vi "asyncAcq_occurenceRef_timeStamp.vi"(0 "reference":refnum<class "OSA.lvclass">, 5 "error in (no error)":errorcluster) -> (14 "duplicate reference":refnum<class "OSA.lvclass">, 15 "new spectrum":bool, 16 "new interferogram":bool, 18 "error":u32, 19 "error out":errorcluster)   [LabVIEW 2010, in "OSA.lvclass"]
doc: "Reads the contents of a <B>Thorlabs_OSA_64</B> object.\n\n[GOOP 1.0]"
uses:
  OSA.lvclass
panel:
  out "timeStamp interferogram":u32
  out "timeStamp spectrum":u32
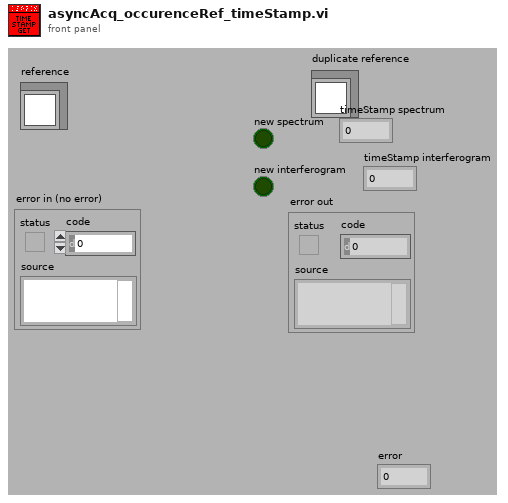
[diagram p1: front panel]
types:
  T1 = typedef "OSA.lvclass/ObjectAttributes.ctl" = cluster{"Stop":bool, "dataType":T2, "spectrometerIdx":u16, "buffer size interferogram":i32, "interferogram":cluster{"new":bool, "plot_x_ min":sgl, "plot_x_max":sgl, "plot_y_min":sgl, "plot_y_max":sgl, "Graph Intrfrgrm":T3, "timeStamp":u32, "signal (%)":dbl, "traces":cluster{"idx":u32, "broadBand":bool, "monoChromatic":bool, "peakToPeakSignal":dbl, "peakToPeakPos":dbl}[], "traces idx last":i32}, "spectrum":cluster{"new":bool, "plot_x_min":sgl, "plot_x_max":sgl, "plot_unit_x":T4, "plot_unit_y":T5, "plot_y_min":sgl, "plot_y_max":sgl, "Graph Spectrum":T3, "timeStamp":u32, "X_VAL_OPTIONS":enum16{"MIN_MAX", "ARRAY"}, "traces":cluster{"idx":u32}[], "traces idx last":i32}, "Thorlabs_OSA_64.lvclass:queue_action.ctlqueue ref":refnum<queue>, "action":T6, "plot zoom step":dbl, "buffer semaphore":T7, "acq stopped":bool, "dataType active":T2, "temperature (degr C)":sgl, "pressure (hPa)":sgl, "rel humidity (%)":sgl, "settings":cluster{"resolution":T8, "sensitivity":T9, "Average":bool, "average nr":u32, "apodisation":T10, "acq delay (ms)":u32, "airMesure":T11, "wmtr on":bool, "intfgrm_smooth_width":u16, "intfgrm_smooth_nrOfPasses":u16, "intfgrm_smooth":T12, "phaseCorrection":T13, "zeroFill":u8, "spectr_smooth":T12, "spectr_smooth_width":u16, "spectr_smooth_nrOfPasses":u16, "resolution (/cm)":sgl, "REF wavelength, (nm)":dbl, "gain_idx":u16, "gainAuto":bool, "gain_relative":dbl, "PD sensitivity mode":T14, "PD senseMode implemented":bool, "SensorTemperature implemented":bool, "SensorPressure implemented":bool, "SensorHumidity implemented":bool}, "peaks position":sgl[], "peaks width":sgl[], "peaks height":sgl[], "peaks max nr":u32, "peaks latest nr":i32, "peaks new":bool, "power":dbl, "power new":bool, "path":string, "wavelength (WNr)":dbl, "wavelength new":bool, "buffer size spectrum":i32, "status":string, "VI reference":refnum<vi>, "funcPointer":u64, "libraryPointer":u64, "singleAcquisition":bool, "coherenceLength (cm)":dbl, "coherenceLength new":bool, "spectrometer model":string, "spectrometer serial nr":string, "peaks thld left":sgl[], "peaks thld right":sgl[], "coherenceLength error (cm)":dbl, "ADC bits":u16, "peaks position centroid":sgl[], "peaks height centroid":sgl[], "OSA series":T15, "channel index spectrum":u16, "spectrometer rangeLow, (/cm)":dbl, "spectrometer rangeHigh, (/cm)":dbl, "channel index interferogram":u16}
  T2 = typedef "OSA.lvclass/acq_dataType.ctl" = enum16{"none", "interferogram", "spectrum"}
  T3 = typedef "OSA.lvclass/graph_intensity.ctl" = refnum<vi>
  T4 = typedef "OSA.lvclass/spectrum_x_unit.ctl" = enum16{"wavenr/cm", "THz", "eV", "nm_air", "nm_vac"}
  T5 = typedef "OSA.lvclass/y_unit.ctl" = enum16{"ADC counts", "dBm pwr absolute", "dBm pwr density", "mW pwr absolute", "mW pwr density"}
  T6 = typedef "OSA.lvclass/queue_action.ctl" = enum16{"none", "stop", "GUI_plotInterferogram", "GUI_plotSpectrum", "GUI_plotInterferogramRescale", "GUI_plotSpectrumRescale", "GUI_plotInterferogramReset", "GUI_plotSpectrumReset", "GUI_plotInterferogramAutoScaleY", "GUI_plotSpectrumAutoScaleY", "GUI_plotInterferogramZoomOut", "GUI_plotSpectrumZoomOut", "GUI_plotInterferogramPane", "GUI_plotSpectrumPane", "GUI_plotInterferogramZoomMouse", "GUI_plotSpectrumZoomMouse", "ENVIRONMENT temperature", "ENVIRONMENT pressure", "MODE_resolution set", "MODE_resolution get", "MODE_sensitivity set", "MODE_sensitivity get", "MODE_PDTemperature set", "MODE_PDTemperature get", "REBOOT/RESET firmware", "ACQASYNC_acquireSingleSpectrum", "ACQASYNC_continuous start", "ACQASYNC_continuous stop\n", "ACQASYNC_get last interferogram", "ACQASYNC_get last spectrum", "ACQASYNC_get last waveNr", "ACQOPT_interferogram smoothing set", "ACQOPT_interferogram smoothing get", "ACQOPT_spectrum smoothing set", "ACQOPT_spectrum smoothing get", "ACQOPT_apodisation type set", "ACQOPT_apodisation type get", "ACQOPT_phase correction type set", "ACQOPT_phase correction type get", "ACQOPT_acqIntervall_set", "ACQOPT_acqIntervall_get", "ACQOPT_average spectrum set", "ACQOPT_average spectrum get", "ACQOPT_rolling average set", "ACQOPT_rolling average get", "ACQOPT_zero fill factor set", "ACQOPT_zero fill factor get", "ACQOPT_cycle counting set", "ACQOPT_cycle counting get", "ACQOPT_air measure option set", "ACQOPT_air measure option get", "ACQOPT_gainLevel auto get", "ACQOPT_gainLevel auto set", "ACQOPT_gainLevel get", "ACQOPT_gainLevel set", "ACQOPT_getAll", "INSTRUMENT_PROPERTY_range_WaveNr_min", "INSTRUMENT_PROPERTY_range_WaveNr_max", "INSTRUMENT_PROPERTY_reference_wavelength_cm^-1", "INSTRUMENT_PROPERTY_samplesPerRefPeriod", "INSTRUMENT_PROPERTY_resolution_waveNrPercm", "INSTRUMENT_PROPERTY_availableGainLevels", "INSTRUMENT_PROPERTY_status", "CONVERT", "ANALYSE_POWER", "ANALYSE_PEAKS", "ANALYSE_WAVELENGTH", "ANALYSE_SPECTRUM", "ANALYSE_INTERFEROGRAM", "ANALYSE_COHERENCE_LENGTH", "MATH", "MATH_power", "MATH_peaks", "FILE", "miscellaneous"}
  T7 = typedef "Semaphore RefNum" = refnum<k1>
  T8 = typedef "OSA.lvclass/resolution.ctl" = enum16{"low", "high"}
  T9 = typedef "OSA.lvclass/sensitivityMode.ctl" = enum16{"low", "low medium", "high medium", "high"}
  T10 = typedef "OSA.lvclass/apodisation.ctl" = enum16{"NONE", "NORTON_BEER_WEAK", "NORTON_BEER_MEDIUM", "NORTON_BEER_STRONG", "TRIANGULAR", "COSINE", "HANN", "HAMMING", "BLACKMANHARRIS3", "BLACKMANHARRIS4", "GAUSSIAN"}
  T11 = typedef "OSA.lvclass/airMeasure.ctl" = enum16{"TEMPERATURE", "PRESSURE"}
  T12 = typedef "OSA20X_misc.lvlib/interferogram_smoothing.ctl" = enum16{"NONE", "BINOMIAL", "SAVITSKY_GOLAY", "FOURIER", "MOVING_AVERAGE", "GAUSSIAN"}
  T13 = typedef "OSA.lvclass/phaseCorrection.ctl" = enum16{"NONE", "MERTZ", "FORMAN", "MERTZ_FILE", "FORMAN_FILE", "FUTURE COMP."}
  T14 = typedef "OSA20X_misc.lvlib/PDTemperatureMode.ctl" = enum16{"cool: better sensitivity/noise floor", "warm: extended wl range"}
  T15 = typedef "OSA.lvclass/OSA_series.ctl" = enum16{"OSA200", "OSA300", "UNKNOWN"}
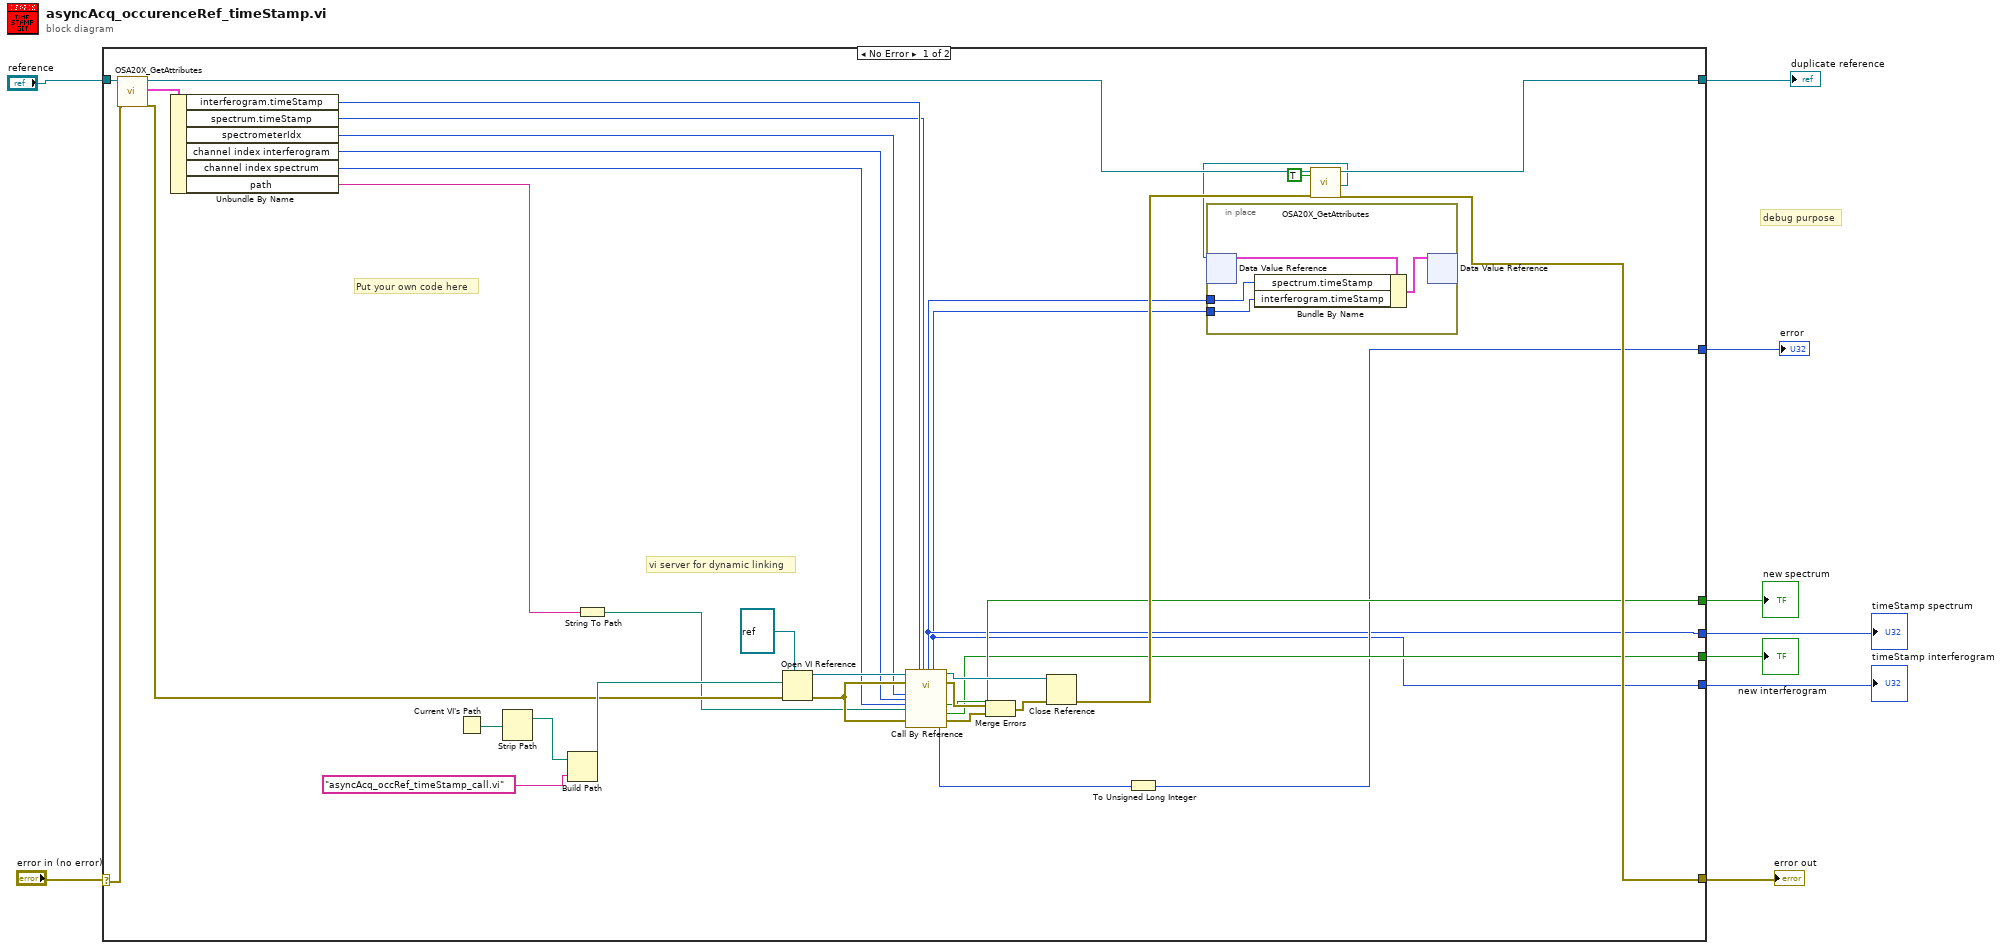
[diagram p0: block diagram]
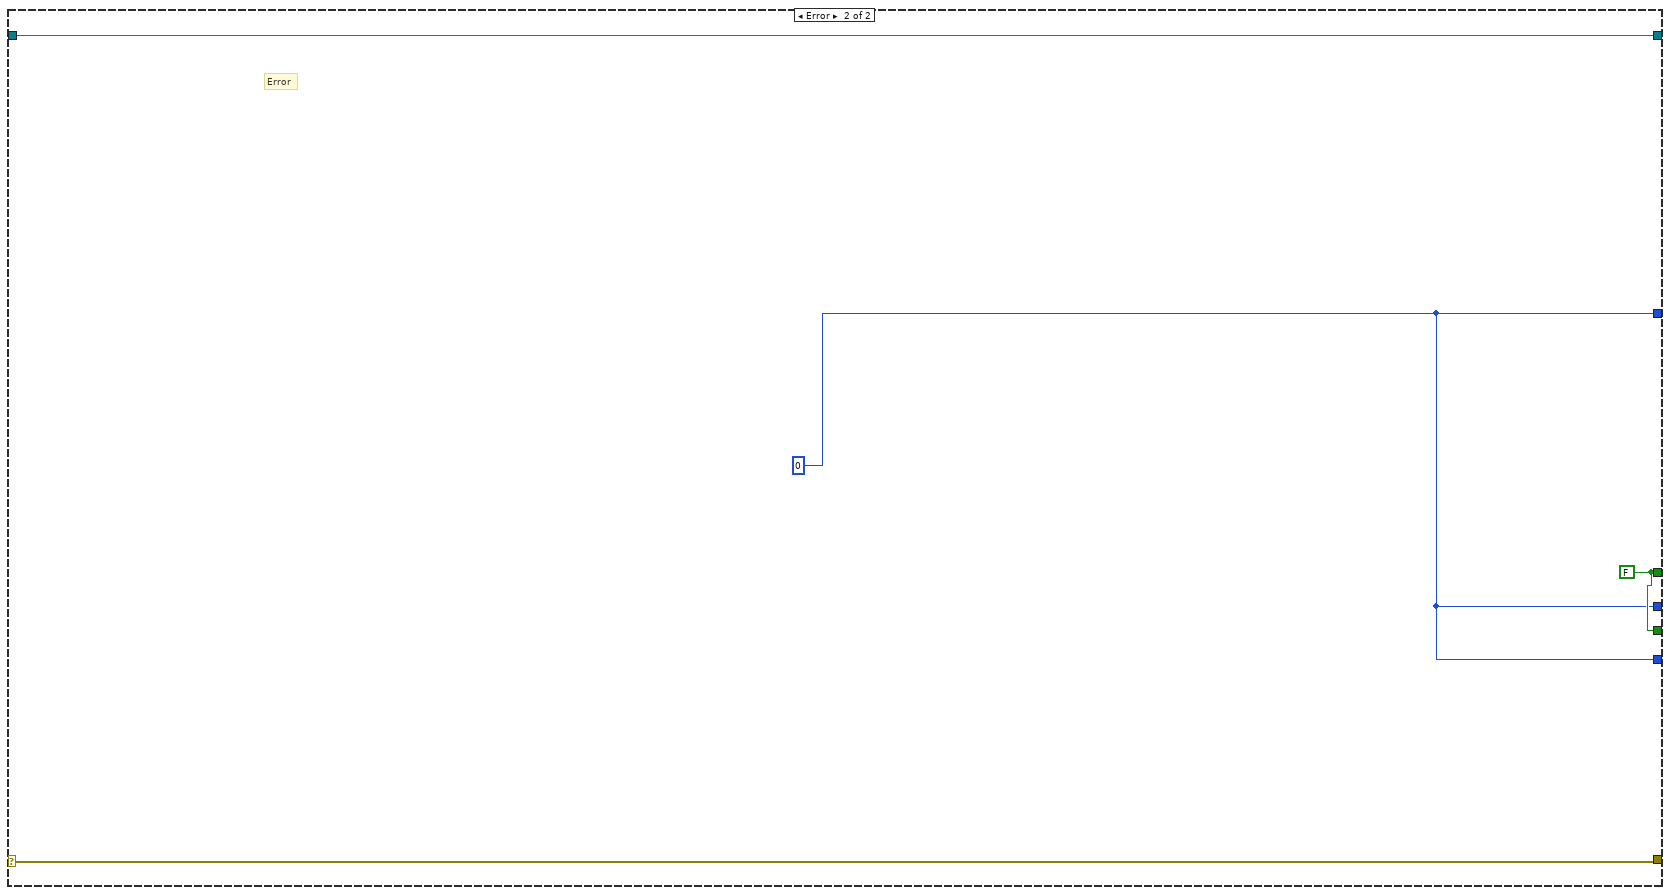
[diagram p2: hidden frame]
diagram:
  # "debug purpose"
  n1 = case shown="No Error" "error in (no error)" {
    selector: "error in (no error)" -> [w42 w50]
    tunnel: [w39 w50] -> w9
    tunnel: "reference" -> [w43 w51]
    tunnel: [w40 w51] -> w6
    tunnel: [w20 w48] -> w5
    tunnel: [w23 w49] -> w4
    tunnel: [w22 w49] -> w3
    tunnel: [w15 w48] -> w2
    tunnel: [w14 w48] -> w1
    frame No Error {
      # "vi server for dynamic linking"
      # "Put your own code here"
      n2 = call "OSA20X_GetAttributes.vi"("reference in"=w43, "error in (no error)"=w42) -> ("reference out"=w41:refnum<class "OSA.lvclass">, "Data"=w17:T1, "error out"=w25:errorcluster)  [unwired: 14 in, 1 out]
      n3 = Unbundle By Name(w17) -> ("interferogram.timeStamp"=w27:u32, "spectrum.timeStamp"=w26:u32, "spectrometerIdx"=w28:u16, "channel index interferogram"=w11:u16, "channel index spectrum"=w10:u16, "path"=w12:string)
      n4 = Current VI's Path() -> (path=w37:path)
      n5 = Strip Path(path=w37) -> (stripped path=w36:path)  [unwired: 1 out]
      n6 = Build Path(base path=w36, name or relative path="asyncAcq_occRef_timeStamp_call.vi") -> (appended path=w34:path)
      n7 = String To Path(string=w12) -> (path=w13:path)
      n8 = Open VI Reference(type specifier VI Refnum (for type only)=refnum<vi> refnum, vi path=w34, error in (no error)=w25) -> (vi reference=w38:refnum<vi>, error out=w32:errorcluster)  [unwired: 3 in]
      n9 = call-by-ref "?"(reference=w38, error in=w32, "spectrIdx"=w28, "channelIdx interferogram"=w11, "channelIdx spectrum"=w10, "FTSLV.dll path"=w13, 5:"error in (no error)"=w32, "timeStamp interferogram"=w27, "timeStamp spectrum"=w26) -> (reference out=w33:refnum<vi>, error out=w30:errorcluster, "timeStamp spectrum latest"=w15:u32, "timeStamp interferogram latest"=w14:u32, "error"=w21:i32, "new spectrum"=w23:bool, "new interferogram"=w22:bool, 19:"error out"=w29:errorcluster)  [unwired: 7 in]
      n10 = Merge Errors(w30, w29) -> (w31:errorcluster)
      n11 = Close Reference(reference=w33, error in (no error)=w31) -> (error out=w24:errorcluster)
      n12 = To Unsigned Long Integer(number=w21) -> (unsigned 32bit integer=w20:u32)
      n13 = call "OSA20X_GetAttributes.vi"("reference in"=w41, "OnlyGetDvrReference(False)"=TRUE, "error in (no error)"=w24) -> ("reference out"=w40:refnum<class "OSA.lvclass">, "DataRef"=w16:refnum<data-value>, "error out"=w39:errorcluster)  [unwired: 13 in, 1 out]
      n14 = in-place {
        in-place-border: w15 -> [w46]
        in-place-border: w14 -> [w45]
        n15 = in-place-dvr #1(w16) -> (w47:T1)  [unwired: 1 out]
        n16 = Bundle By Name(cluster=w47, "spectrum.timeStamp"=w46, "interferogram.timeStamp"=w45) -> (w44:T1)
        n17 = in-place-dvr #1(w44) -> ()  [unwired: 2 out]
      }
    }
    frame Error {
      w48 = u16 0 ("spectrIdx")
      w49 = FALSE
      # "Error"
    }
  }
  "error out" <- w9
  "duplicate reference" <- w6
  "error" <- w5
  "new spectrum" <- w4
  "new interferogram" <- w3
  "timeStamp spectrum" <- w2
  "timeStamp interferogram" <- w1
